vi "Write Forward Drive Config.vi"(8 "error in (no error)":errorcluster, 10 "Forward Drive Config":T1={"Left Motors with Encoders"=refnum, "Right Motors with Encoders"=refnum, "Encoder Control"=TRUE}, 11 "Forward Drive in":refnum<class "Forward Drive.lvclass">) -> (0 "error out":errorcluster, 3 "Forward Drive out":refnum<class "Forward Drive.lvclass">)   [LabVIEW 2014, in "Forward Drive.lvlib" / "Forward Drive.lvclass"]
uses:
  Forward Drive.lvclass
  Forward Drive Config.ctl
  Motor with Encoders/Motors with Encoders Class/Motors with Encoders.lvclass
  Forward Drive.lvclass/Forward Drive.ctl
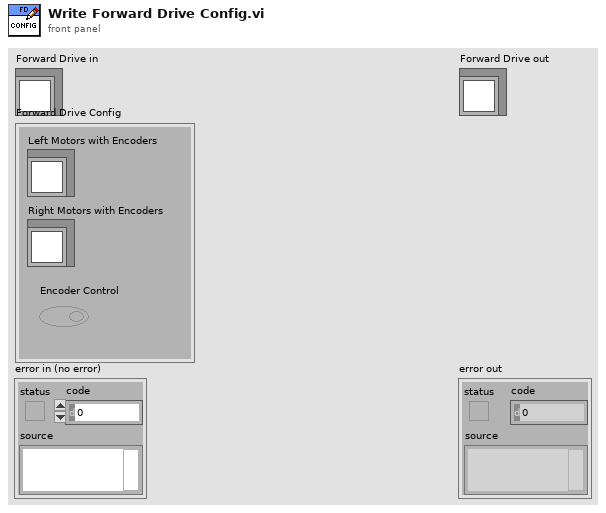
[diagram p1: front panel]
types:
  T1 = typedef "Forward Drive.lvlib/Forward Drive.lvclass/Forward Drive Config.ctl" = cluster{"Left Motors with Encoders":refnum<class "Motors with Encoders.lvclass">, "Right Motors with Encoders":refnum<class "Motors with Encoders.lvclass">, "Encoder Control":bool}
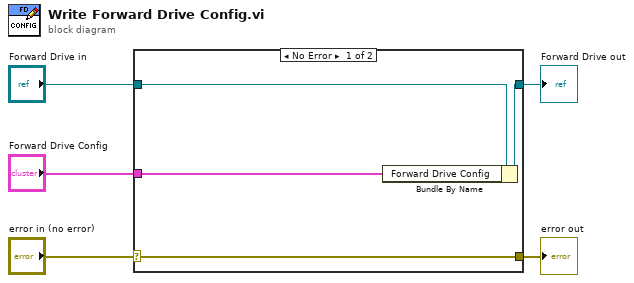
[diagram p0: block diagram]
diagram:
  n1 = case shown="No Error" "error in (no error)" {
    selector: "error in (no error)" -> [w9 w10]
    tunnel: [w9 w10] -> w4
    tunnel: [w7 w11] -> w2
    tunnel: "Forward Drive in" -> [w8 w11]
    tunnel: "Forward Drive Config" -> [w6 _]
    frame No Error {
      n2 = Bundle By Name(cluster=w8, "Forward Drive Config"=w6) -> (w7:refnum<class "Forward Drive.lvclass">)
    }
    frame Error {
    }
  }
  "error out" <- w4
  "Forward Drive out" <- w2
